vi "teste.vi"() -> ()   [LabVIEW 2022 SP3]
panel:
  out "Var":bool
  out "current time":timestamp
  in  "Stop":bool
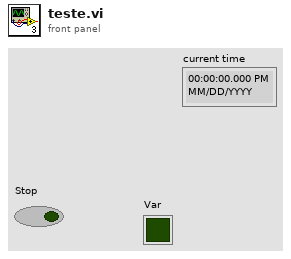
[diagram p1: front panel]
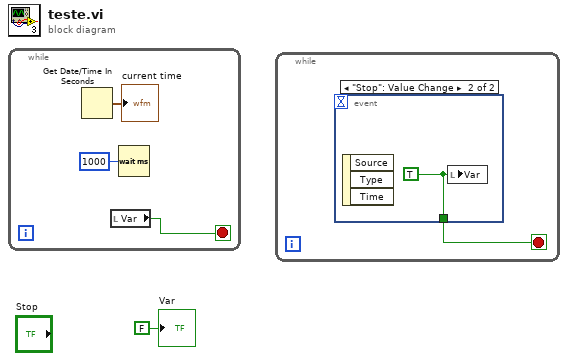
[diagram p0: block diagram]
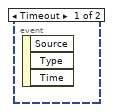
[diagram p2: hidden frame]
diagram:
  n1 = while {
    stop <- w2 stop-if-true
    n2 = Get Date/Time In Seconds() -> (seconds since 1Jan1904=→"current time":timestamp)
    n3 = local read "Var"() -> (w2:bool)
    n4 = Wait (ms)(milliseconds to wait=u32 1000) -> ()  [unwired: 1 out]
  }
  n5 = while {
    stop <- w5 stop-if-true
    n6 = event shown="[1] \"Stop\": Value Change" {
      selector: _ -> [_ _]
      dyn-events: _ -> [_ _]
      timeout: _ -> [_ _]
      tunnel: [_ w6] -> w5
      event Timeout {
        n7 = event-data() -> ()  [unwired: 1 in, 3 out]
      }
      event "Stop": Value Change {
        w6 = TRUE ("Var")
        n8 = event-data() -> ()  [unwired: 1 in, 3 out]
        n9 = local write "Var"(w6) -> ()
      }
    }
  }
  "Var" <- FALSE ("Var")
